vi "Read Connection Test.vi"() -> ()   [LabVIEW 2009]
panel:
  out "x = y?":bool
  out "substring 2":string
  out "number":dbl
  out "substring":string
  in  "Read":bool
  in  "stop":bool
  out "data out":string
  in  "data in":string
  out "error out":errorcluster
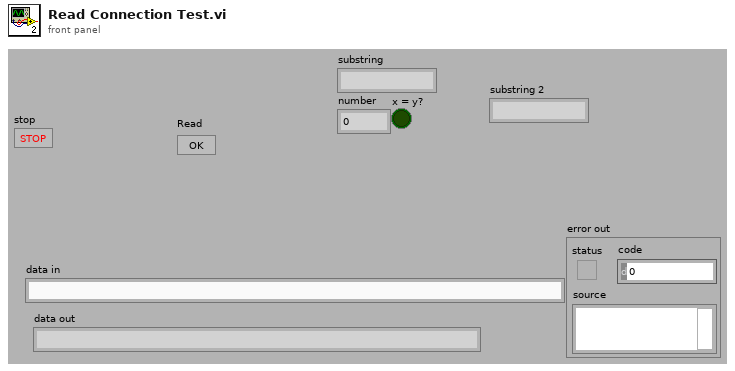
[diagram p1: front panel]
types:
  T1 = enum16{"Standard", "Buffered", "CRLF", "Immediate"}
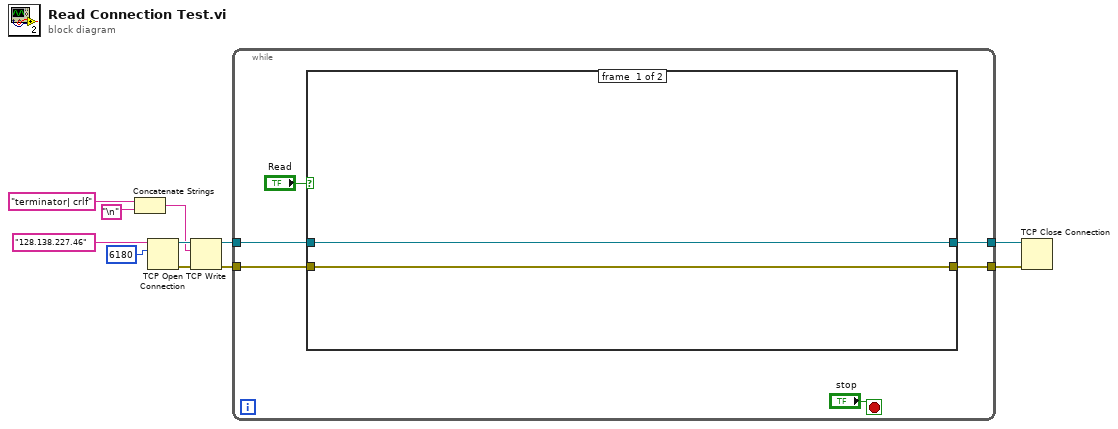
[diagram p0: block diagram]
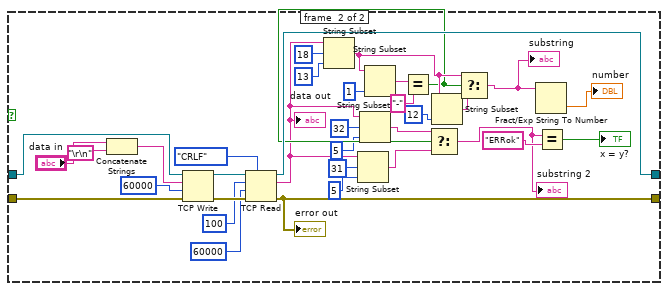
[diagram p2: hidden frame]
diagram:
  n1 = Concatenate Strings("terminator| crlf" ("data in"), "\n") -> (w6:string)
  n2 = TCP Open Connection(address="128.138.227.46", remote port or service name=u16 6180) -> (connection ID=w9:refnum<k5>, error out=w5:errorcluster)  [unwired: 3 in]
  n3 = TCP Write(connection ID=w9, data in=w6, error in (no error)=w5) -> (connection ID out=w4:refnum<k5>, error out=w3:errorcluster)  [unwired: 1 in, 1 out]
  n4 = while {
    tunnel: w4 -> [w16]
    tunnel: w3 -> [w15]
    tunnel: [w14] -> w2
    tunnel: [w13] -> w1
    stop <- "stop" stop-if-true
    n5 = case shown="True" "Read" {
      tunnel: w16 -> [w19 w47]
      tunnel: w15 -> [w18 w46]
      tunnel: [w19 w45] -> w14
      tunnel: [w18 w44] -> w13
      frame #0 {
      }
      frame #1 {
        n6 = Concatenate Strings("data in", "\r\n") -> (w49:string)
        n7 = TCP Write(connection ID=w47, data in=w49, error in (no error)=w46, 9:60000 ("timeout ms (25000)")) -> (connection ID out=w53:refnum<k5>, error out=w52:errorcluster)  [unwired: 1 out]
        n8 = TCP Read(connection ID=w53, bytes to read=100, error in (no error)=w52, 7:T1."CRLF" ("mode (standard)"), 9:60000 ("timeout ms (25000)")) -> (connection ID out=w45:refnum<k5>, data out=w23:string, error out=w44:errorcluster)
        "error out" <- w44
        "data out" <- w23
        n9 = String Subset(string=w23, offset (0)=18, length (rest)=13 ("length (rest)")) -> (substring=w30:string)
        n10 = String Subset(string=w23, offset (0)=31, length (rest)=5 ("length (rest)")) -> (substring=w25:string)
        n11 = String Subset(string=w23, offset (0)=32, length (rest)=5 ("length (rest)")) -> (substring=w22:string)
        n12 = String Subset(string=w30, length (rest)=1 ("length (rest)")) -> (substring=w32:string)  [unwired: 1 in]
        n13 = Equal?(x=w32, y="-") -> (x = y?=w26:bool)
        n14 = Select(t=w22, s=w26, f=w25) -> (s? t:f=w20:string)
        "substring 2" <- w20
        n15 = String Subset(string=w30, length (rest)=12 ("length (rest)")) -> (substring=w28:string)  [unwired: 1 in]
        n16 = Select(t=w30, s=w26, f=w28) -> (s? t:f=w29:string)
        "substring" <- w29
        n17 = Fract/Exp String To Number(string=w29) -> (number=→"number":dbl)  [unwired: 3 in, 1 out]
        n18 = Equal?(x=w20, y="ERRok") -> (x = y?=→"x = y?":bool)
      }
    }
  }
  n19 = TCP Close Connection(connection ID=w2, error in (no error)=w1) -> ()  [unwired: 1 in, 2 out]
